vi "data buffer.vi"(0 "voltage data":sgl[][](array[numeric]) format="%.4f", 1 "action":enum16{"write", "read", "clear"}(ring), 2 "scan rate (Hz)":dbl format="%.2f", 3 "max buffer":i32=1000) -> (4 "time at AI start":dbl format="%.2f", 5 "more data":bool, 6 "data out":T1 {"seconds since 1904" format="%<%I:%M:%S %p\n%m/%d/%Y>T"; "voltage data" format="%.4f"}, 7 "buffer size":i32, 8 "got data":bool, 9 "lost data":bool)   [LabVIEW 2015]
uses:
  data w time.ctl
panel:
  out "reads":i32
  out "writes":i32
  # "scan #"
  # "channel"
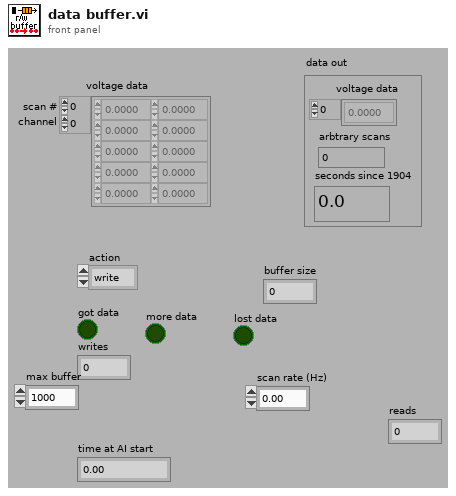
[diagram p1: front panel]
types:
  T1 = typedef "data w time.ctl" = cluster{"voltage data":sgl[], "seconds since 1904":dbl, "arbtrary scans":u32}
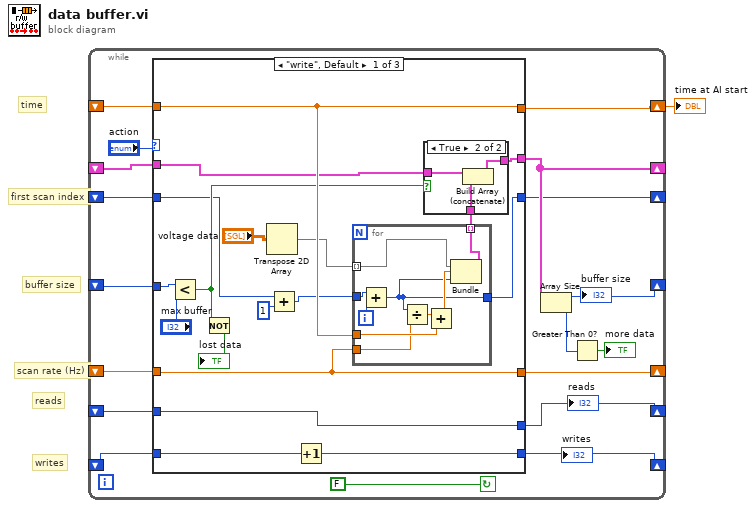
[diagram p0: block diagram]
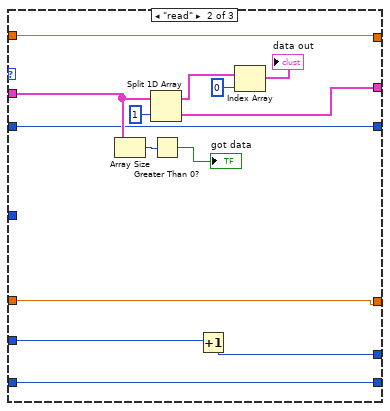
[diagram p3: hidden frame]
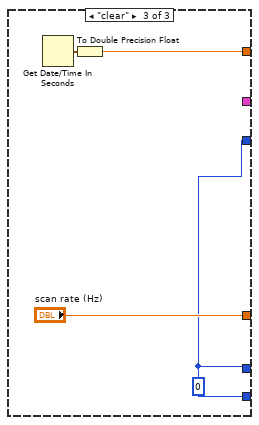
[diagram p4: hidden frame]
diagram:
  # "buffer size"
  # "time"
  # "writes"
  # "reads"
  # "scan rate (Hz)"
  # "first scan index"
  n1 = while {
    shift-right: [w15] -> _
    shift-left: _ -> [w18]
    shift-right: [w13] -> _
    shift-left: _ -> [w14]
    shift-right: [w11] -> _
    shift-left: _ -> [w12]
    shift-right: [w8] -> w1
    shift-left: _ -> [w7]
    shift-right: [w6] -> _
    shift-left: _ -> [w5]
    shift-right: [w10] -> _
    shift-left: _ -> [w4]
    shift-right: [w3] -> _
    shift-left: _ -> [w2]
    stop <- FALSE continue-if-true
    n2 = case shown="\"write\", Default" "action" {
      tunnel: [w36 w61 _] -> w15
      tunnel: w18 -> [w30 w56 _]
      tunnel: w14 -> [w35 w55 _]
      tunnel: [w34 w55 w65] -> w13
      tunnel: [w33 w53 w65] -> w11
      tunnel: w12 -> [w33 w54 _]
      tunnel: [w32 w52 w67] -> w8
      tunnel: w7 -> [w32 w52 _]
      tunnel: [w31 w51 "scan rate (Hz)"] -> w6
      tunnel: w5 -> [w31 w51 _]
      tunnel: w4 -> [w29 _ _]
      tunnel: [w23 w50 w65] -> w3
      tunnel: w2 -> [w20 w50 _]
      frame "write", Default {
        n3 = Less?(x=w29, y="max buffer") -> (x < y?=w25:bool)
        n4 = Not(x=w25) -> (.not. x?=→"lost data":bool)
        n5 = Transpose 2D Array(2D array="voltage data") -> (transposed array=w19:sgl[][])
        n6 = Add(x=w20, y=u32 1) -> (x+y=w21:u32)
        n7 = Increment(x=w35) -> (x+1=w34:i32)
        n8 = for {
          tunnel: [w49] -> w26 mode=indexing
          tunnel: w19 -> [w42] mode=indexing
          tunnel: w21 -> [w48]
          tunnel: w32 -> [w44]
          tunnel: w31 -> [w43]
          tunnel: [w41] -> w23
          i -> [w47]
          n9 = Add(x=w48, y=w47) -> (x+y=w41:u32)
          n10 = Divide(x=w41, y=w43) -> (x/y=w46:dbl)
          n11 = Add(x=w46, y=w44) -> (x+y=w45:dbl)
          n12 = Bundle(w42, w45, w41) -> (w49:cluster{sgl[], dbl, u32})  [unwired: 1 in]
        }
        n13 = case shown="True" w25 {
          tunnel: [w37 w40] -> w36
          tunnel: w30 -> [_ w39]
          tunnel: w26 -> [w37 w38]
          frame False {
          }
          frame True {
            n14 = Build Array (concatenate)(w39, w38) -> (w40:cluster{sgl[], dbl, u32}[])
          }
        }
      }
      frame "read" {
        n15 = Array Size(array=w56) -> (size(s)=w57:i32)
        n16 = Split 1D Array(array=w56, index=1) -> (first subarray=w60:cluster{sgl[], dbl, u32}[], second subarray=w61:cluster{sgl[], dbl, u32}[])
        n17 = Greater Than 0?(x=w57) -> (x > 0?=→"got data":bool)
        n18 = Increment(x=w54) -> (x+1=w53:i32)
        n19 = Index Array(array=w60, index=0) -> (element=→"data out":cluster{sgl[], dbl, u32})
      }
      frame "clear" {
        w65 = 0
        n20 = Get Date/Time In Seconds() -> (seconds since 1Jan1904=w64:timestamp)
        n21 = To Double Precision Float(number=w64) -> (double precision float=w67:dbl)
      }
    }
    "writes" <- w13
    "reads" <- w11
    n22 = Array Size(array=w15) -> (size(s)=w10:i32)
    "buffer size" <- w10
    n23 = Greater Than 0?(x=w10) -> (x > 0?=→"more data":bool)
  }
  "time at AI start" <- w1
